vi "FTW-ScripterStep-Wait-Core_Process.vi"(0 "FTW Actor Instance Configuration":string="{\n  \"Identity\": \"ActorName\",\n  \"InboxAddress\": \"inproc://*\",\n  \"LoggerAddress\": \"\",\n  \"My Data\": false,\n  \"Publisher URI\": \"inproc://*\",\n  \"Subscriber URIs\": \"\",\n  \"Refresh Period\": 2\n}", 11 "ErrorIn":errorcluster) -> (15 "Error":errorcluster)   [LabVIEW 2015, in "FTW-ScripterStep-Wait-Core.lvclass"]
uses:
  FTW-ScripterStep-Wait-Core.lvclass
  FTW-ScripterStep-Wait-Core.lvclass/FTW-ScripterStep-Wait-Core.ctl
  source/actor/Instance/FTW-ActorInstance.lvclass/FTW-ActorInstance.ctl
  source/actor/JobSequencer/FTW-SEQ-Current.vi
  source/actor/Message/Base/FTW-Message.lvclass
  source/actor/Instance/FTW-ActorInstance.lvclass
  source/actor/Message/Request/FTW-Message-IncomingRequest.lvclass
  source/actor/Publisher/FTW-Publisher.lvclass
panel:
  # "#TODO\nhide controls for a GUI"
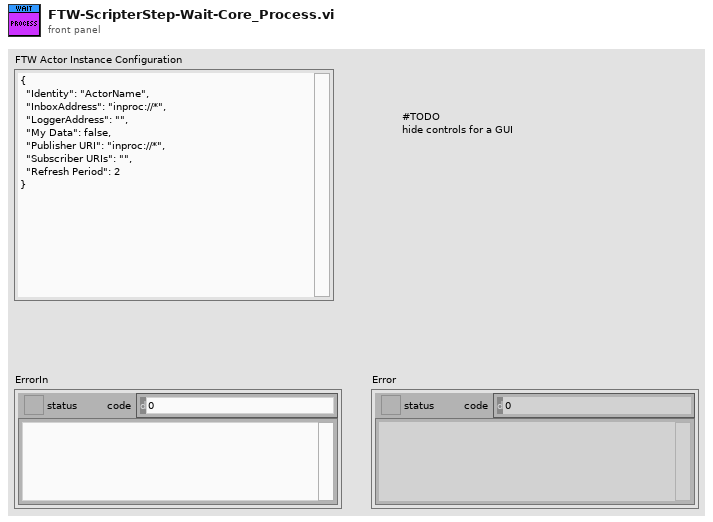
[diagram p1: front panel]
types:
  T1 = cluster{"Incoming Requests":refnum<event-registration>, "Local Messages":refnum<event-registration>}
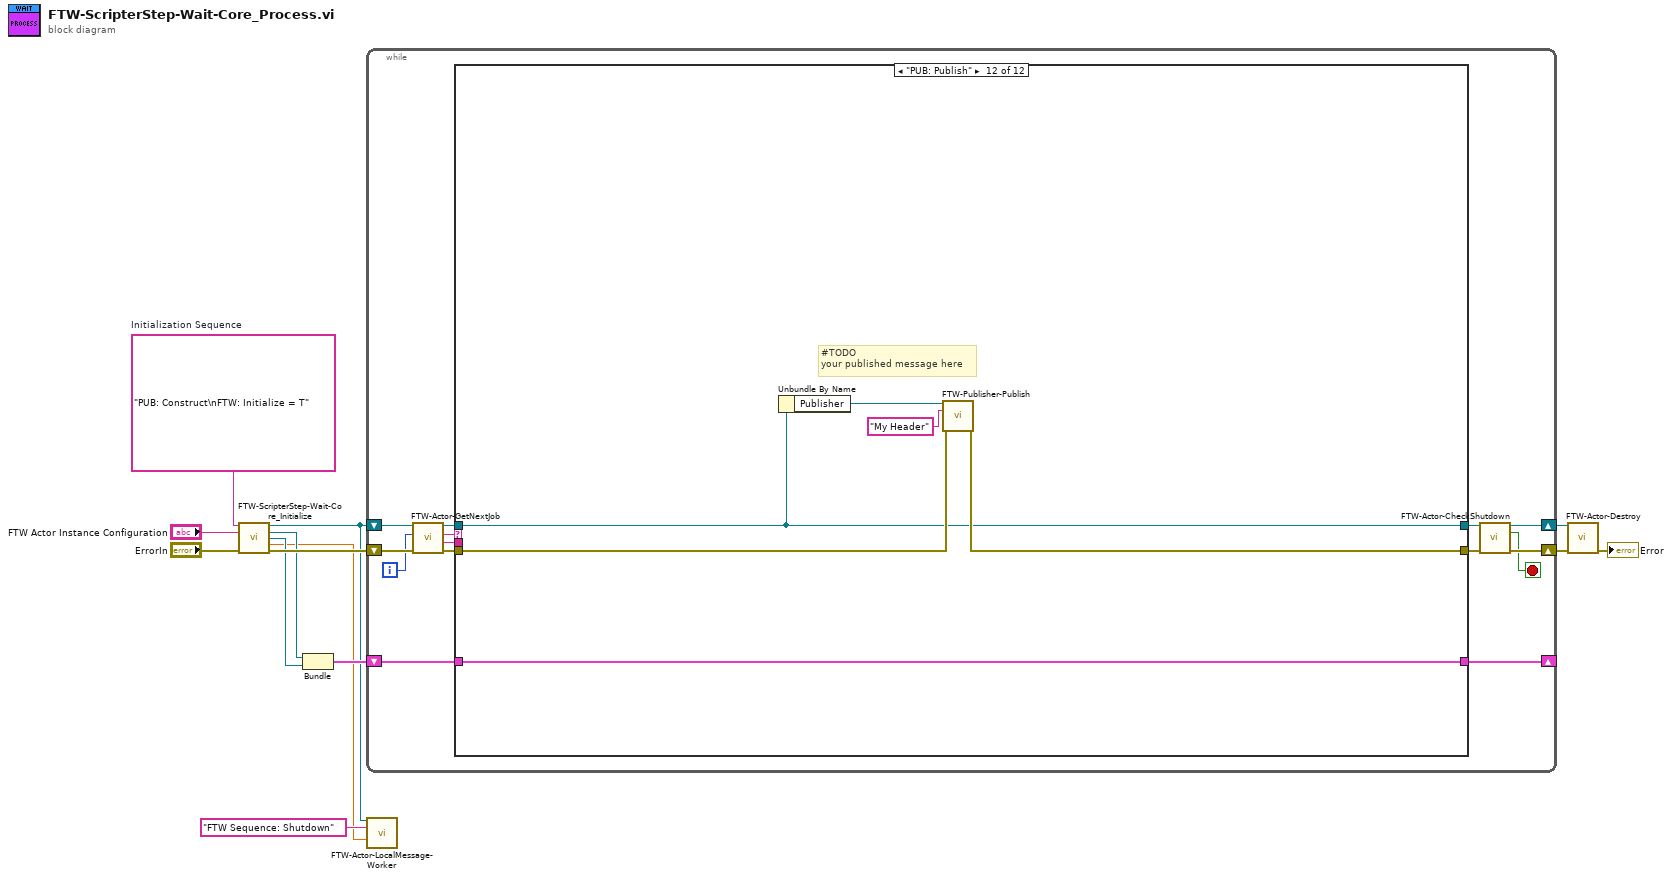
[diagram p0: block diagram]
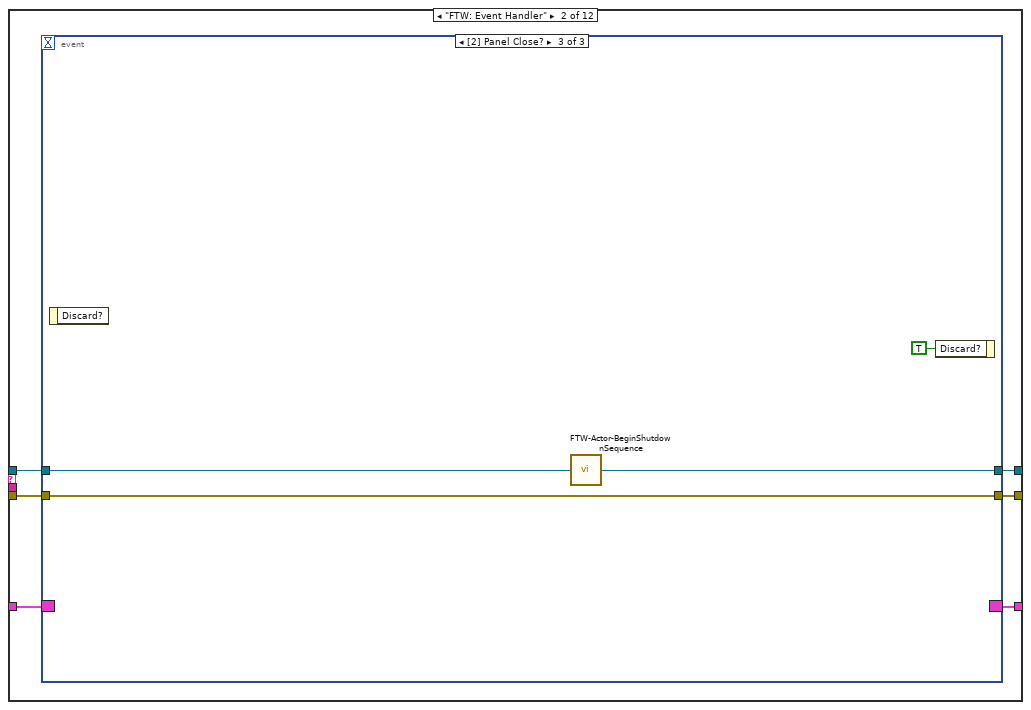
[diagram p3: hidden frame]
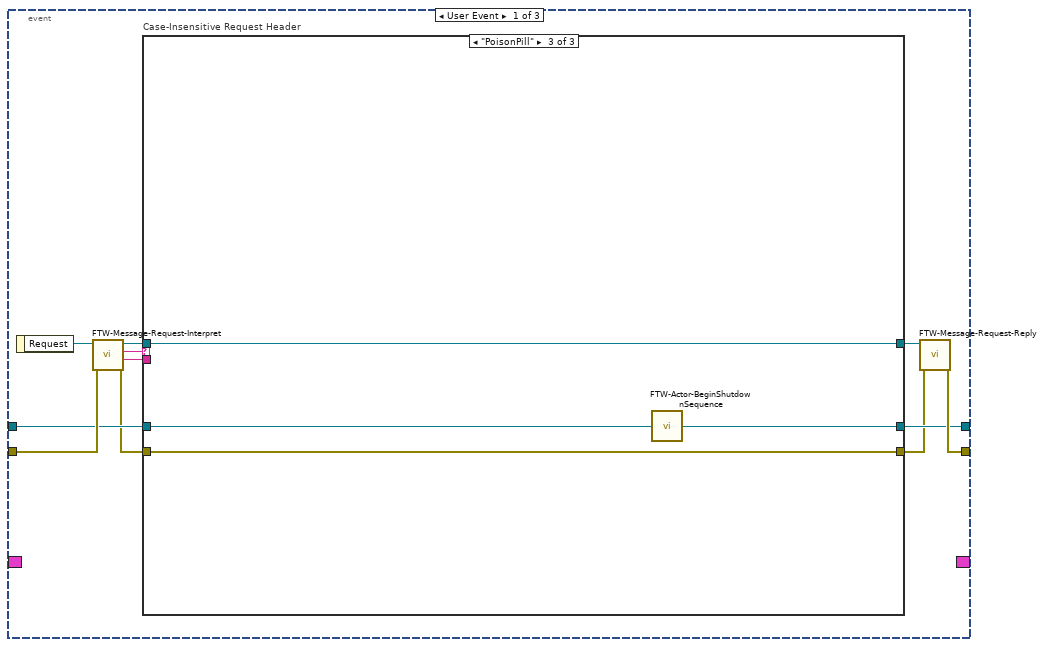
[diagram p4: hidden frame]
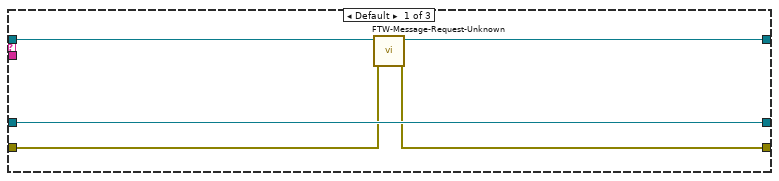
[diagram p5: hidden frame]
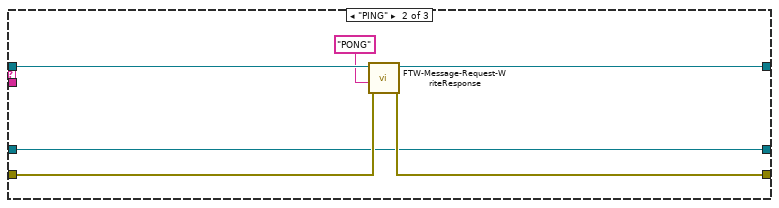
[diagram p6: hidden frame]
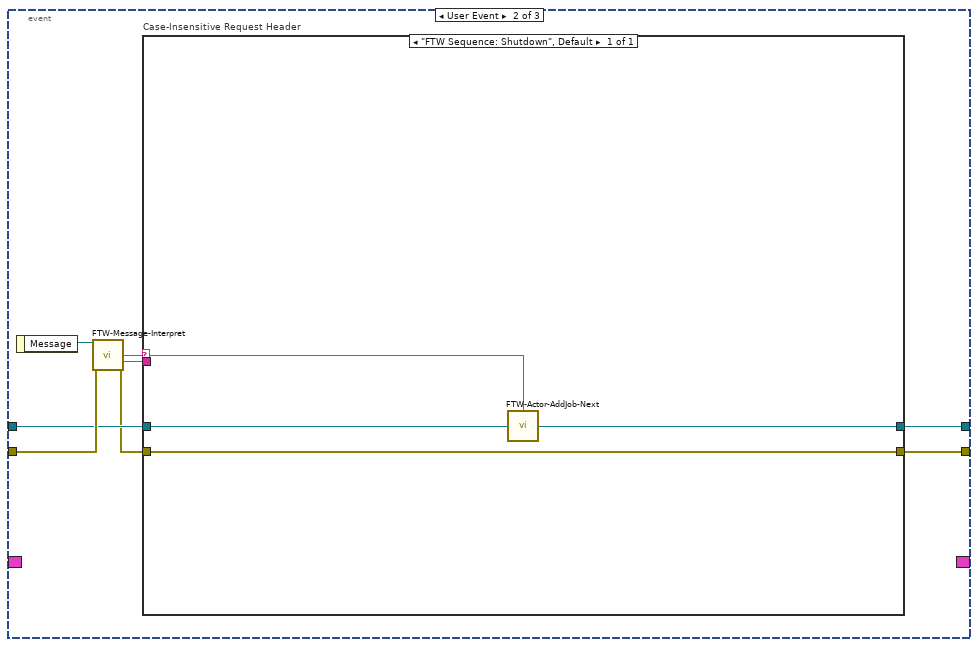
[diagram p7: hidden frame]
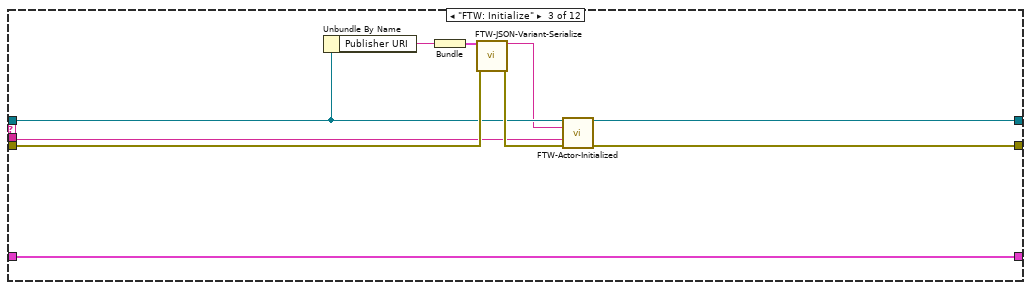
[diagram p8: hidden frame]
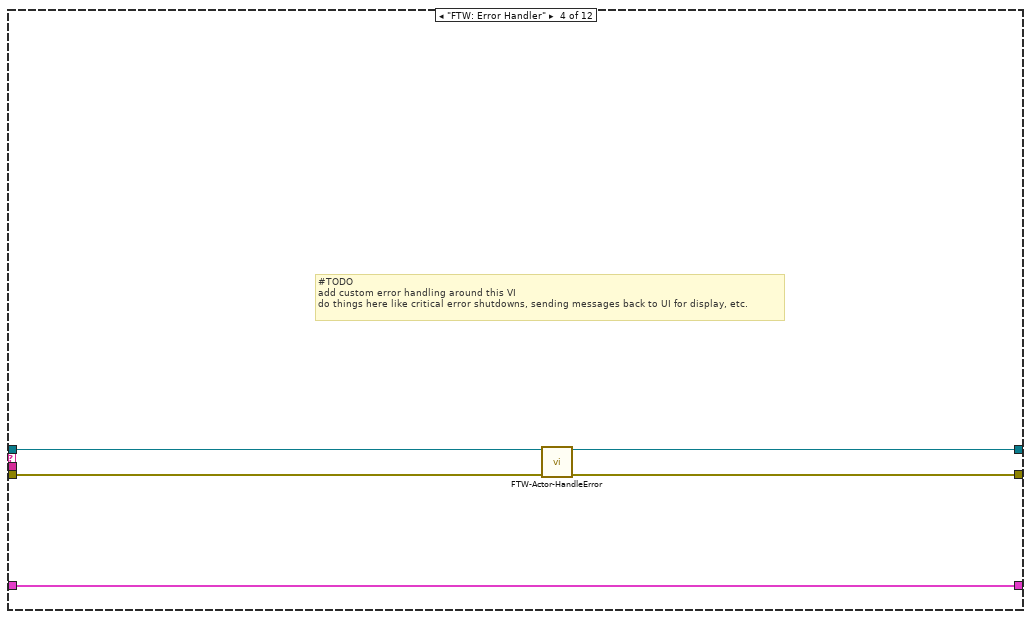
[diagram p9: hidden frame]
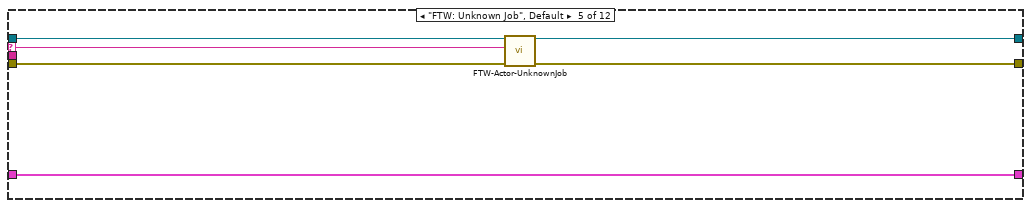
[diagram p10: hidden frame]
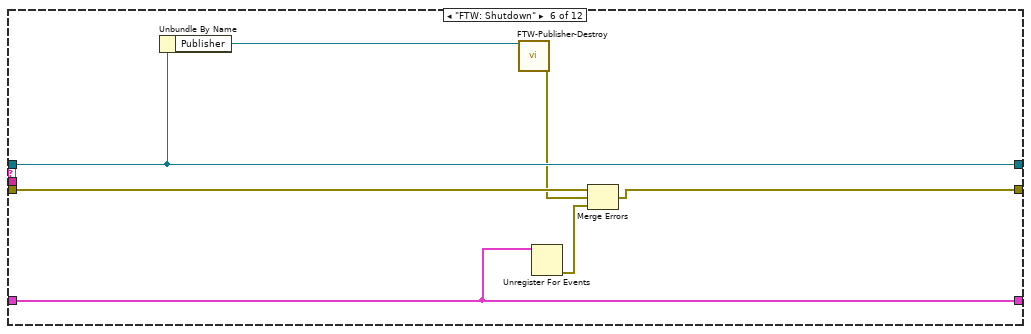
[diagram p11: hidden frame]
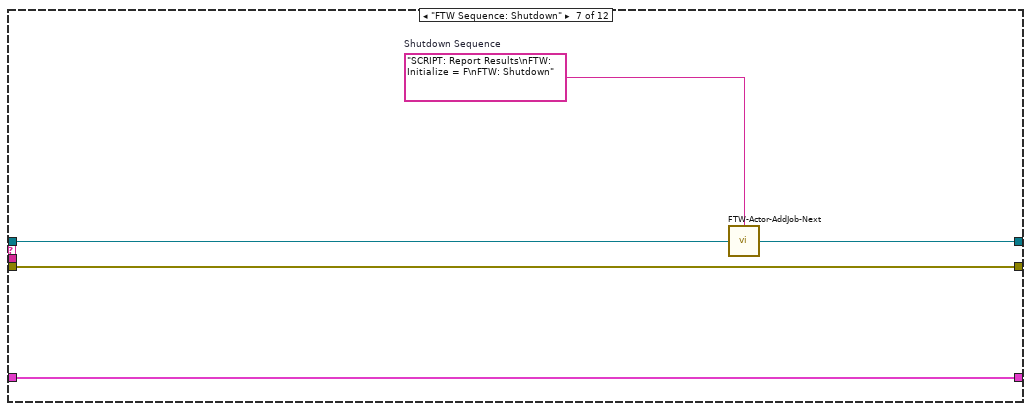
[diagram p12: hidden frame]
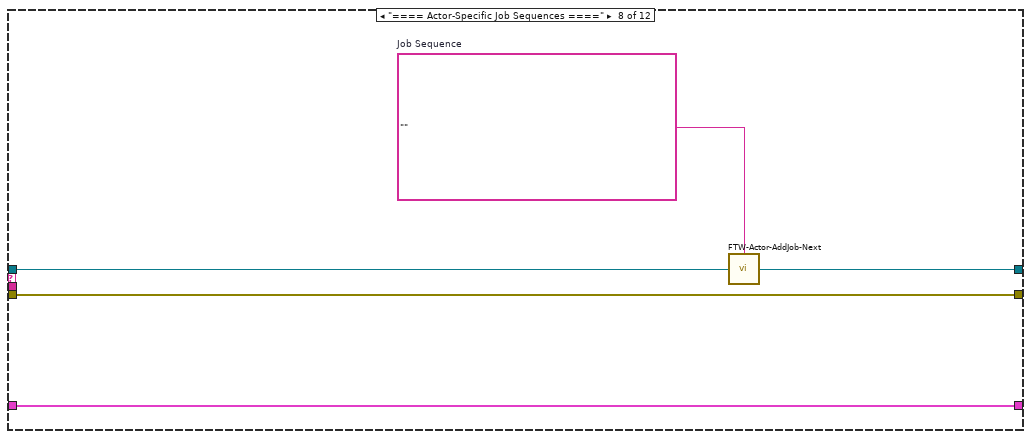
[diagram p13: hidden frame]
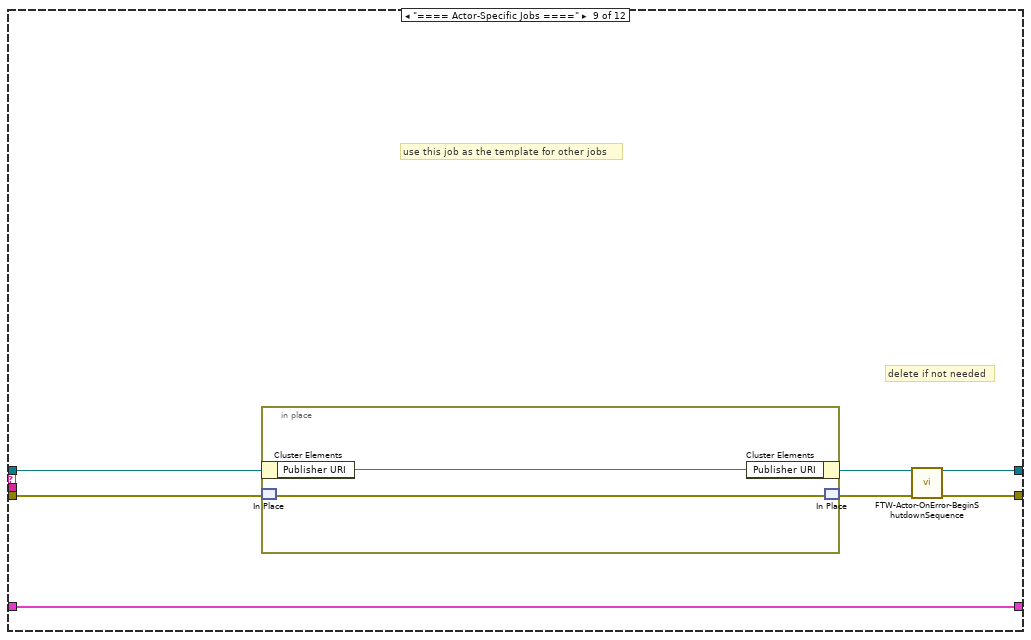
[diagram p14: hidden frame]
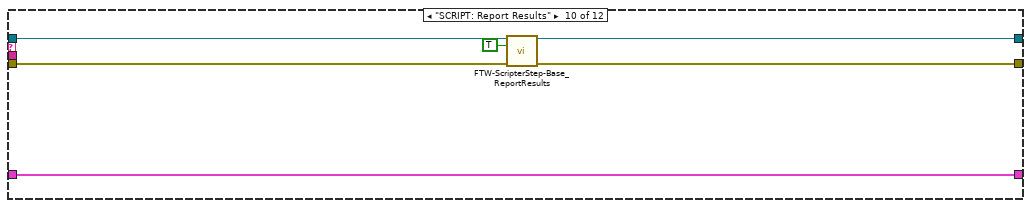
[diagram p15: hidden frame]
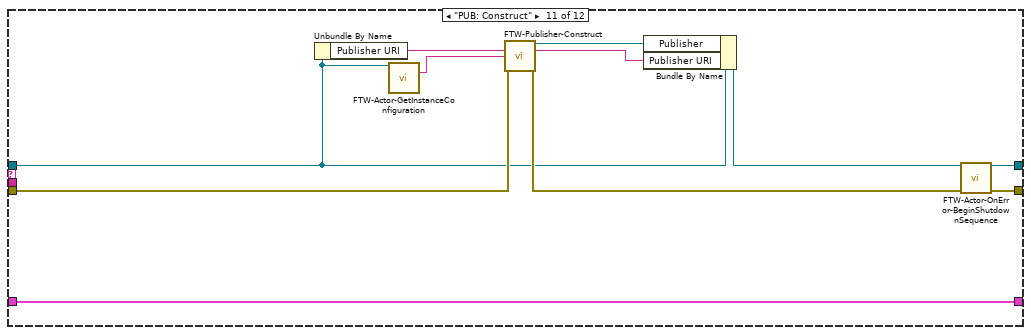
[diagram p16: hidden frame]
diagram:
  w9 = "PUB: Construct\nFTW: Initialize = T"  # Initialization Sequence
  n1 = call "FTW-ScripterStep-Wait-Core_Initialize.vi"("Initialization Sequence"=w9, "FTW Actor Instance Configuration"="FTW Actor Instance Configuration", "error in (no error)"="ErrorIn") -> ("Actor Template-Core out"=w2:refnum<class "FTW-ScripterStep-Wait-Core.lvclass">, "Incoming Requests"=w5:refnum<event-registration>, "Local Messages"=w4:refnum<event-registration>, "Wait Time"=w1:dbl, "error out"=w10:errorcluster)  [unwired: 8 in]
  n2 = Bundle("Incoming Requests"=w5, "Local Messages"=w4) -> (w7:T1)  [unwired: 1 in]
  n3 = while {
    shift-right: [w17] -> w12
    shift-left: w10 -> [w24]
    shift-right: [w14] -> _
    shift-left: w7 -> [w27]
    shift-right: [w19] -> w13
    shift-left: w2 -> [w26]
    i -> [w15]
    stop <- w16 stop-if-true
    n4 = call "FTW-Actor-GetNextJob.vi"("error in"=w24, "Jobs Performed"=w15, "FTW Actor Instance"=w26) -> ("error out"=w23:errorcluster, "Job Data"=w21:string, "Job Name"=w22:string, "FTW Actor Instance out"=w25:refnum<class "FTW-ScripterStep-Wait-Core.lvclass">)  [unwired: 5 in]
    n5 = case shown="\"PUB: Publish\"" w22 {
      selector: w22 -> [_ _ _ _ w94 _ _ _ _ _ _ _]
      tunnel: [w29 w36 w84 w89 w97 w105 w110 w115 w119 w127 w138 w146] -> w18
      tunnel: w23 -> [w29 w35 w88 w91 w98 w106 w110 w115 w122 w130 w140 w147]
      tunnel: w27 -> [w30 w31 w86 w93 w99 w103 w111 w116 w123 w131 w142 w148]
      tunnel: [w30 w34 w86 w93 w99 w103 w111 w116 w123 w131 w142 w148] -> w14
      tunnel: w21 -> [_ _ w81 _ _ _ _ _ _ _ _ _]
      tunnel: [w28 w33 w85 w90 w95 w102 w108 w113 w117 w128 w136 w145] -> w20
      tunnel: w25 -> [w28 w32 w83 w92 w96 w102 w109 w114 w120 w129 w133 w145]
      frame "==== Featherweight Framework Jobs ====" {
      }
      frame "FTW: Event Handler" {
        n6 = event shown="[2] Panel Close?" {
          selector: w31 -> [_ _ _]
          dyn-events: [_ _ _] -> w34
          timeout: _ -> [_ _ _]
          tunnel: [w46 w65 w77] -> w36
          tunnel: w35 -> [w45 w69 w77]
          tunnel: [w40 w66 w75] -> w33
          tunnel: w32 -> [w44 w68 w76]
          event User Event {
            n7 = event-data() -> ("Request"=w47:refnum<class "FTW-Message-IncomingRequest.lvclass">)  [unwired: 1 in]
            n8 = call "FTW-Message-Request-Interpret.vi"("error in"=w45, "FTW Incoming Request"=w47) -> ("error out"=w43:errorcluster, "Request Body"=w37:string, "Request Header"=w41:string, "FTW Incoming Request out"=w42:refnum<class "FTW-Message-IncomingRequest.lvclass">)  [unwired: 6 in]
            n9 = case "Case-Insensitive Request Header" shown="\"PoisonPill\"" w41 {
              tunnel: [w50 w56 w61] -> w39
              tunnel: w43 -> [w51 w57 w61]
              tunnel: [w52 w55 w62] -> w40
              tunnel: w44 -> [w52 w55 w60]
              tunnel: w42 -> [w49 w58 w59]
              tunnel: [w48 w54 w59] -> w38
              tunnel: w37 -> [_ _ _]
              frame Default {
                n10 = call "FTW-Message-Request-Unknown.vi"("error in"=w51, "FTW Incoming Request"=w49) -> ("error out"=w50:errorcluster, "FTW Incoming Request Out"=w48:refnum<class "FTW-Message-IncomingRequest.lvclass">)  [unwired: 8 in]
              }
              frame "PING" {
                n11 = call "FTW-Message-Request-WriteResponse.vi"("error in"=w57, "Response Body"="PONG" ("Response Header"), "FTW Incoming Request"=w58) -> ("error out"=w56:errorcluster, "FTW Incoming Request out"=w54:refnum<class "FTW-Message-IncomingRequest.lvclass">)  [unwired: 7 in]
              }
              frame "PoisonPill" {
                n12 = call "FTW-Actor-BeginShutdownSequence.vi"("FTW Actor Instance"=w60) -> ("FTW Actor Instance out"=w62:refnum<class "FTW-ScripterStep-Wait-Core.lvclass">)  [unwired: 3 in]
              }
            }
            n13 = call "FTW-Message-Request-Reply.vi"("FTW: Reply Error"=w39, "FTW Incoming Request"=w38) -> ("error out"=w46:errorcluster)  [unwired: 8 in, 1 out]
          }
          event User Event {
            n14 = event-data() -> ("Message"=w70:refnum<class "FTW-Message.lvclass">)  [unwired: 1 in]
            n15 = call-dynamic "FTW-Message-Interpret.vi"("FTW Message"=w70, "error in"=w69) -> ("Message Header"=w64:string, "Message Body"=w63:string, "error out"=w67:errorcluster)  [unwired: 9 in, 2 out]
            n16 = case "Case-Insensitive Request Header" shown="\"FTW Sequence: Shutdown\", Default" w64 {
              selector: w64 -> [w71]
              tunnel: [w73] -> w65
              tunnel: w67 -> [w73]
              tunnel: [w72] -> w66
              tunnel: w68 -> [w74]
              tunnel: w63 -> [_]
              frame "FTW Sequence: Shutdown", Default {
                n17 = call "FTW-Actor-AddJob-Next.vi"("Add Next in Job Queue"=w71, "FTW Actor Instance"=w74) -> ("FTW Actor Instance out"=w72:refnum<class "FTW-ScripterStep-Wait-Core.lvclass">)  [unwired: 2 in]
              }
            }
          }
          event Panel Close? {
            n18 = event-data() -> ()  [unwired: 1 in, 1 out]
            n19 = call "FTW-Actor-BeginShutdownSequence.vi"("FTW Actor Instance"=w76) -> ("FTW Actor Instance out"=w75:refnum<class "FTW-ScripterStep-Wait-Core.lvclass">)  [unwired: 3 in]
            n20 = event-data("Discard?"=TRUE) -> ()  [unwired: 1 in, 1 out]
          }
        }
      }
      frame "FTW: Initialize" {
        n21 = Unbundle By Name(w83) -> ("Publisher URI"=w82:string)
        n22 = Bundle("Publisher URI"=w82) -> (w80:cluster{"Publisher URI":string})  [unwired: 1 in]
        n23 = call "FTW-JSON-Variant-Serialize.vi"("Variant"=w80, "error in"=w88) -> ("JSON String"=w79:string, "error out"=w87:errorcluster)  [unwired: 12 in]
        n24 = call-dynamic "FTW-Actor-Initialized.vi"("FTW Actor Instance"=w83, "Initialized Response"=w79, "Positive Init?"=w81, "error in"=w87) -> ("FTW Actor Instance out"=w85:refnum<class "FTW-ScripterStep-Wait-Core.lvclass">, "error out"=w84:errorcluster)  [unwired: 10 in]
      }
      frame "FTW: Error Handler" {
        # "#TODO\nadd custom error handling around this VI\ndo things here like critical error shutdowns, sending messages back to UI for display, etc."
        n25 = call-dynamic "FTW-Actor-HandleError.vi"("FTW Actor Instance"=w92, "error in"=w91) -> ("FTW Actor Instance out"=w90:refnum<class "FTW-ScripterStep-Wait-Core.lvclass">, "error out"=w89:errorcluster)  [unwired: 10 in, 2 out]
      }
      frame "FTW: Unknown Job", Default {
        n26 = call-dynamic "FTW-Actor-UnknownJob.vi"("FTW Actor Instance"=w96, "Unknown Job"=w94, "error in"=w98) -> ("FTW Actor Instance out"=w95:refnum<class "FTW-ScripterStep-Wait-Core.lvclass">, "error out"=w97:errorcluster)  [unwired: 11 in]
      }
      frame "FTW: Shutdown" {
        n27 = Unbundle By Name(w102) -> ("Publisher"=w101:refnum<class "FTW-Publisher.lvclass">)
        n28 = call "FTW-Publisher-Destroy.vi"("FTW-Publisher In"=w101) -> ("error out"=w100:errorcluster)  [unwired: 14 in]
        n29 = Unregister For Events(event registration refnum=w103) -> (error out=w104:errorcluster)  [unwired: 1 in]
        n30 = Merge Errors(w106, w100, w104) -> (w105:errorcluster)
      }
      frame "FTW Sequence: Shutdown" {
        w107 = "SCRIPT: Report Results\nFTW: Initialize = F\nFTW: Shutdown"  # Shutdown Sequence
        n31 = call "FTW-Actor-AddJob-Next.vi"("Add Next in Job Queue"=w107, "FTW Actor Instance"=w109) -> ("FTW Actor Instance out"=w108:refnum<class "FTW-ScripterStep-Wait-Core.lvclass">)  [unwired: 2 in]
      }
      frame "==== Actor-Specific Job Sequences ====" {
        w112 = ""  # Job Sequence
        n32 = call "FTW-Actor-AddJob-Next.vi"("Add Next in Job Queue"=w112, "FTW Actor Instance"=w114) -> ("FTW Actor Instance out"=w113:refnum<class "FTW-ScripterStep-Wait-Core.lvclass">)  [unwired: 2 in]
      }
      frame "==== Actor-Specific Jobs ====" {
        # "delete if not needed"
        # "use this job as the template for other jobs"
        n33 = in-place {
          n34 = in-place-cluster #1(w120) -> ("Publisher URI"=w124:string)
          n35 = in-place-match #2(w122) -> (w125:errorcluster)
          n36 = in-place-cluster #1("Publisher URI"=w124) -> (w118:refnum<class "FTW-ScripterStep-Wait-Core.lvclass">)
          n37 = in-place-match #2(w125) -> (w121:errorcluster)
        }
        n38 = call-dynamic "FTW-Actor-OnError-BeginShutdownSequence.vi"("FTW Actor Instance"=w118, "error in"=w121) -> ("FTW Actor Instance out"=w117:refnum<class "FTW-ScripterStep-Wait-Core.lvclass">, "error out"=w119:errorcluster)  [unwired: 12 in]
      }
      frame "SCRIPT: Report Results" {
        n39 = call-dynamic "FTW-ScripterStep-Base_ReportResults.vi"("FTW-ScripterStep-Base In"=w129, "Passed"=TRUE, "error in (no error)"=w130) -> ("FTW-ScripterStep-Base Out"=w128:refnum<class "FTW-ScripterStep-Wait-Core.lvclass">, "error out"=w127:errorcluster)  [unwired: 11 in]
      }
      frame "PUB: Construct" {
        n40 = Unbundle By Name(w133) -> ("Publisher URI"=w134:string)
        n41 = call "FTW-Actor-GetInstanceConfiguration.vi"("FTW Actor Instance"=w133) -> ("Identity"=w132:string)  [unwired: 12 in, 2 out]
        n42 = call "FTW-Publisher-Construct.vi"("Address"=w134, "Identity"=w132, "error in"=w140) -> ("FTW-Publisher Out"=w141:refnum<class "FTW-Publisher.lvclass">, "Actual Address"=w135:string, "error out"=w139:errorcluster)  [unwired: 10 in]
        n43 = Bundle By Name(cluster=w133, "Publisher"=w141, "Publisher URI"=w135) -> (w137:refnum<class "FTW-ScripterStep-Wait-Core.lvclass">)
        n44 = call-dynamic "FTW-Actor-OnError-BeginShutdownSequence.vi"("FTW Actor Instance"=w137, "error in"=w139) -> ("FTW Actor Instance out"=w136:refnum<class "FTW-ScripterStep-Wait-Core.lvclass">, "error out"=w138:errorcluster)  [unwired: 12 in]
      }
      frame "PUB: Publish" {
        # "#TODO\nyour published message here"
        n45 = Unbundle By Name(w145) -> ("Publisher"=w144:refnum<class "FTW-Publisher.lvclass">)
        n46 = call "FTW-Publisher-Publish.vi"("FTW-Publisher In"=w144, "Header"="My Header", "error in"=w147) -> ("error out"=w146:errorcluster)  [unwired: 11 in, 1 out]
      }
    }
    n47 = call "FTW-Actor-CheckShutdown.vi"("FTW Actor Instance"=w20, "error in"=w18) -> ("FTW Actor Instance out"=w19:refnum<class "FTW-ScripterStep-Wait-Core.lvclass">, "Shutdown?"=w16:bool, "error out"=w17:errorcluster)  [unwired: 11 in]
  }
  n48 = call-dynamic "FTW-Actor-LocalMessage-Worker.vi"("FTW-ActorInstance In"=w2, "Message Header"="FTW Sequence: Shutdown", "Send Rate"=w1) -> ()  [unwired: 13 in]
  n49 = call-dynamic "FTW-Actor-Destroy.vi"("FTW Actor Instance"=w13, "error in"=w12) -> ("error out"=→"Error":errorcluster)  [unwired: 13 in]
